vi "TestStep.vi"(7 "StrInit":string, 8 "error in":errorcluster caption="错误输入（无错误）", 9 "ParaIn":T2={"kCanBaud"=12, "DeviceType"=3, "DevInd"=0, "间隔延时"=0, "ID1(Hex)"="00000182", "DataIN1(Hex)"="000007d100000000", "DataRec1(Hex)"="000007d100000000", "ID2(Hex)"="00000182", "DataIN2(Hex)"="000007d100000000", "DataRec2(Hex)"="000007d100000000"} {"DeviceType" items=["PCI-CAN200"=7, "USB-CAN"=2, "USB-CAN200"=3]; "kCanBaud" items=["250k bps"=10, "10k bps"=2, "5k bps"=1, "50k bps"=5, "40k bps"=4, "20k bps"=3, "80k bps"=6, "100k bps"=7, "125k bps"=8, "200k bps"=9, "400k bps"=11, "500k bps"=12, "666k bps"=13, "800k bps"=14, "1000k bps"=15]}, 10 "ComStr":refnum<vi>, 11 "ComIn":refnum<visa-resource-name>) -> (0 "error out":errorcluster caption="错误输出", 1 "OK?":bool, 2 "通信？":bool, 3 "ComOut":refnum<visa-resource-name>, 4 "Time":u32, 5 "StrOut":string)   [LabVIEW 2013]
uses:
  USBCAN/DevType.ctl
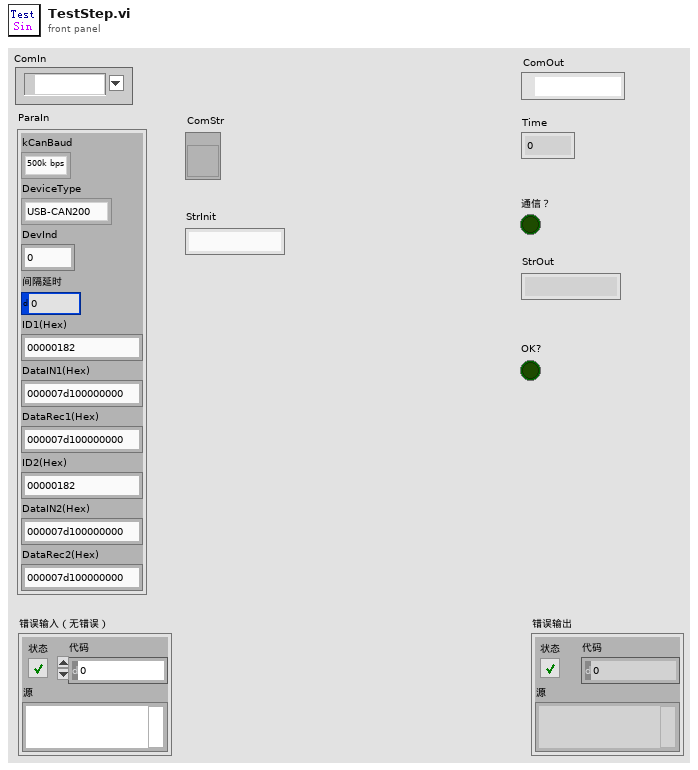
[diagram p1: front panel]
types:
  T1 = typedef "DevType.ctl" = u16
  T2 = cluster{"kCanBaud":u8, "DeviceType":T1, "DevInd":u16, "间隔延时":u32, "ID1(Hex)":string, "DataIN1(Hex)":string, "DataRec1(Hex)":string, "ID2(Hex)":string, "DataIN2(Hex)":string, "DataRec2(Hex)":string}
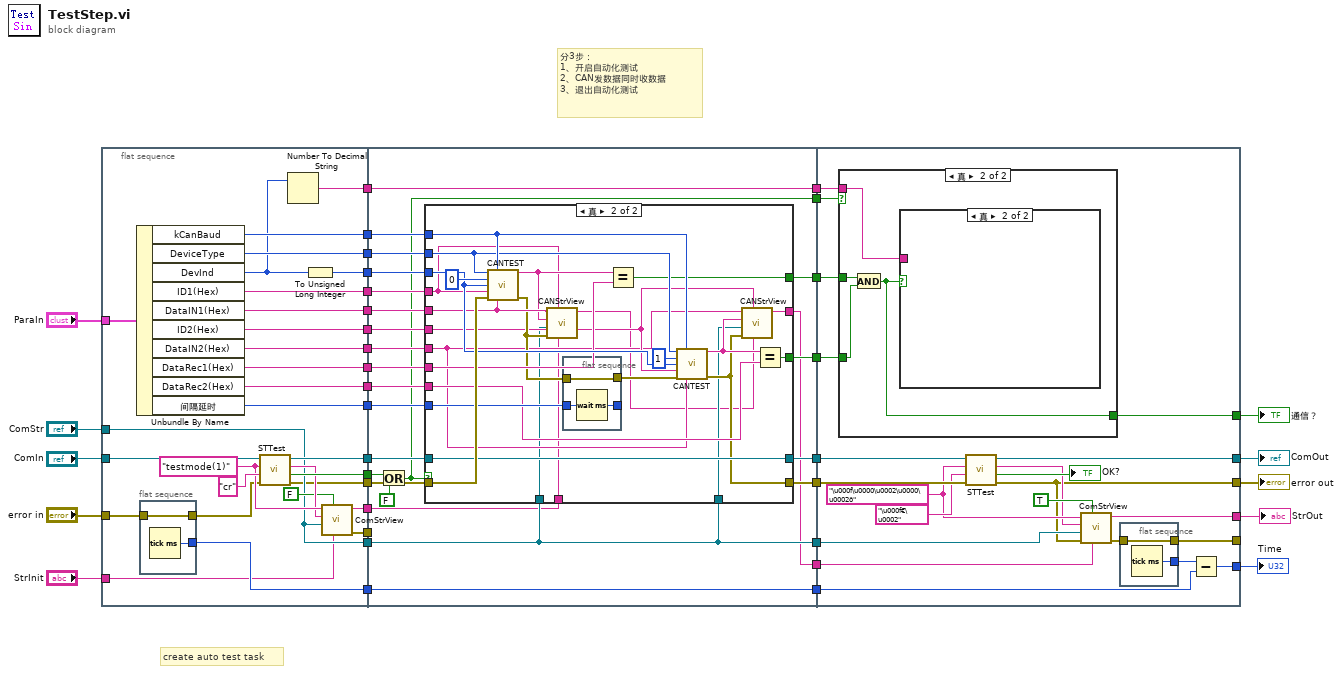
[diagram p0: block diagram]
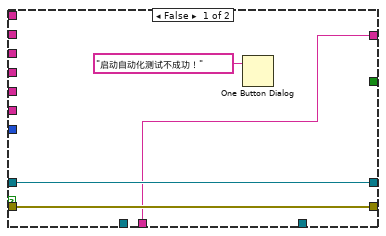
[diagram p2: hidden frame]
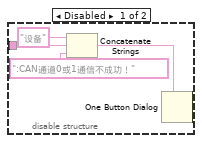
[diagram p5: hidden frame]
diagram:
  # "create auto test task"
  # "分3步：\n1、开启自动化测试\n2、CAN发数据同时收数据\n3、退出自动化测试"
  n1 = flat-sequence {
    tunnel: "ComIn" -> [w65]
    tunnel: "error in" -> [w41]
    tunnel: [w63] -> w35
    tunnel: [w38] -> w34
    tunnel: [w62] -> w33
    tunnel: "ParaIn" -> [w61]
    tunnel: [w60] -> w31
    tunnel: [w59] -> w30
    tunnel: [w49] -> w29
    tunnel: [w58] -> w28
    tunnel: [w57] -> w27
    tunnel: [w56] -> w26
    tunnel: [w55] -> w25
    tunnel: [w54] -> w24
    tunnel: [w53] -> w23
    tunnel: [w52] -> w22
    tunnel: [w50] -> w14
    tunnel: "ComStr" -> [w43]
    tunnel: [w46] -> w10
    tunnel: [w45] -> w9
    tunnel: [w43] -> w8
    tunnel: [w40] -> w6
    tunnel: "StrInit" -> [w39]
    tunnel: w35 -> [w79]
    tunnel: w34 -> [w91]
    tunnel: w33 -> [w72]
    tunnel: w31 -> [w87]
    tunnel: w30 -> [w86]
    tunnel: w29 -> [w85]
    tunnel: w28 -> [w89]
    tunnel: w27 -> [w84]
    tunnel: w26 -> [w90]
    tunnel: w25 -> [w83]
    tunnel: w24 -> [w88]
    tunnel: w23 -> [w82]
    tunnel: w22 -> [w81]
    tunnel: [w78] -> w21
    tunnel: [w80] -> w20
    tunnel: [w71] -> w18
    tunnel: [w77] -> w17
    tunnel: [w76] -> w16
    tunnel: [w75] -> w15
    tunnel: w14 -> [w75]
    tunnel: w10 -> [w69]
    tunnel: w9 -> [_]
    tunnel: w8 -> [w74]
    tunnel: [w74] -> w7
    tunnel: w6 -> [w70]
    tunnel: [w70] -> w5
    tunnel: [w68] -> w3
    tunnel: w21 -> [w146]
    tunnel: w20 -> [w145]
    tunnel: [w144] -> w13
    tunnel: [w125] -> w19
    tunnel: w18 -> [w143]
    tunnel: w17 -> [w142]
    tunnel: w16 -> [w141]
    tunnel: w15 -> [w140]
    tunnel: [w139] -> w12
    tunnel: [w133] -> w2
    tunnel: w7 -> [w132]
    tunnel: [w130] -> _
    tunnel: w5 -> [w128]
    tunnel: [w127] -> w4
    tunnel: w3 -> [w126]
    frame #0 {
      w48 = "testmode(1)" ("CMDIn")
      n2 = Unbundle By Name(w61) -> ("kCanBaud"=w60:u8, "DeviceType"=w59:T1, "DevInd"=w51:u16, "ID1(Hex)"=w56:string, "DataIN1(Hex)"=w58:string, "ID2(Hex)"=w57:string, "DataIN2(Hex)"=w55:string, "DataRec1(Hex)"=w53:string, "DataRec2(Hex)"=w52:string, "间隔延时"=w54:u32)
      n3 = flat-sequence {
        tunnel: [w67] -> w42
        tunnel: w41 -> [w67]
        tunnel: [w66] -> w40
        frame #0 {
          n4 = Tick Count (ms)() -> (millisecond timer value=w66:u32)
        }
      }
      n5 = call "STTest.vi"("error in"=w42, "React"="cr", "CMDIn"=w48, "ComIn"=w65) -> ("error out"=w38:errorcluster, "OK?"=w62:bool, "ReactStr"=w47:string, "ComOut"=w63:refnum<visa-resource-name>)  [unwired: 4 in]
      n6 = Number To Decimal String(number=w51) -> (decimal integer string=w50:string)  [unwired: 1 in]
      n7 = To Unsigned Long Integer(number=w51) -> (unsigned 32bit integer=w49:u32)
      n8 = call "ComStrView.vi"("StrInit"=w39, "Hex？"=FALSE, "ComConn"=w43, "ReactStrIn"=w47, "CMDIn"=w48) -> ("error out"=w45:errorcluster, "连接字符串显示"=w46:string)  [unwired: 5 in]
    }
    frame #1 {
      n9 = Or(x=w72, y=FALSE) -> (x .or. y?=w71:bool)
      n10 = case shown="真" w71 {
        tunnel: w91 -> [w95 w121]
        tunnel: w90 -> [_ w106]
        tunnel: w89 -> [_ w108]
        tunnel: w88 -> [_ w119]
        tunnel: w87 -> [_ w117]
        tunnel: w86 -> [_ w116]
        tunnel: w85 -> [_ w114]
        tunnel: w84 -> [_ w104]
        tunnel: w83 -> [_ w103]
        tunnel: w82 -> [_ w113]
        tunnel: w81 -> [_ w112]
        tunnel: [w95 w101] -> w80
        tunnel: w79 -> [w94 w111]
        tunnel: [w94 w111] -> w78
        tunnel: [_ w110] -> w77
        tunnel: [_ w109] -> w76
        tunnel: w74 -> [_ w100]
        tunnel: w74 -> [_ w99]
        tunnel: w69 -> [w92 w98]
        tunnel: [w92 w96] -> w68
        frame False {
          n11 = One Button Dialog(message="启动自动化测试不成功！" ("消息")) -> ()  [unwired: 1 in, 1 out]
        }
        frame True {
          n12 = call "CANTEST.vi"("DeviceType"=w116, "kCanBaud"=w117, "CANChannel"=u32 0, "DevInd"=w114, "ID(Hex 高位有效)"=w106, "错误输入"=w121, "Data Input(Hex)"=w108) -> ("帧数据"=w107:string, "错误输出"=w105:errorcluster)  [unwired: 5 in, 2 out]
          n13 = call "CANStrView.vi"("StrInit"=w98, "ID"=w106, "error in"=w105, "CANStrView"=w100, "DataRec"=w107, "DataTrans"=w108) -> ("连接显示"=w97:string)  [unwired: 4 in, 1 out]
          n14 = flat-sequence {
            tunnel: w105 -> [w122]
            tunnel: w119 -> [w124]
            tunnel: [w123] -> _
            tunnel: [w122] -> w118
            frame #0 {
              n15 = Wait (ms)(milliseconds to wait=w124) -> (millisecond timer value=w123:u32)
            }
          }
          n16 = Equal?(x=w107, y=w113) -> (x = y?=w110:bool)
          n17 = call "CANTEST.vi"("DeviceType"=w116, "kCanBaud"=w117, "CANChannel"=u32 1, "DevInd"=w114, "ID(Hex 高位有效)"=w104, "错误输入"=w118, "Data Input(Hex)"=w103) -> ("帧数据"=w102:string, "错误输出"=w101:errorcluster)  [unwired: 5 in, 2 out]
          n18 = call "CANStrView.vi"("StrInit"=w97, "ID"=w104, "error in"=w101, "CANStrView"=w99, "DataRec"=w102, "DataTrans"=w103) -> ("连接显示"=w96:string)  [unwired: 4 in, 1 out]
          n19 = Equal?(x=w102, y=w112) -> (x = y?=w109:bool)
        }
      }
    }
    frame #2 {
      w136 = "\u000f\u0000\u0002\u0000\u0002ð"
      n20 = case shown="真" w143 {
        tunnel: w142 -> [_ w152]
        tunnel: w141 -> [_ w151]
        tunnel: w140 -> [_ w150]
        tunnel: [_ w149] -> w139
        frame False {
        }
        frame True {
          n21 = And(x=w152, y=w151) -> (x .and. y?=w149:bool)
          n22 = case shown="真" w149 {
            tunnel: w150 -> [w153 _]
            frame False {
              n23 = disable-structure shown="启用" {
                disable-tunnel: w153 -> [w156 _]
                frame Disabled {
                  n24 = Concatenate Strings("设备", w156, ":CAN通道0或1通信不成功！") -> (w154:string)
                  n25 = One Button Dialog(message=w154) -> ()  [unwired: 1 in, 1 out]
                }
                frame Enabled {
                }
              }
            }
            frame True {
            }
          }
        }
      }
      n26 = call "STTest.vi"("error in"=w145, "React"="\u000f€\u0002", "CMDIn"=w136, "ComIn"=w146) -> ("error out"=w125:errorcluster, "OK?"=→"OK?":bool, "ReactStr"=w134:string, "ComOut"=w144:refnum<visa-resource-name>)  [unwired: 4 in]
      n27 = call "ComStrView.vi"("StrInit"=w126, "Hex？"=TRUE, "error in"=w125, "ComConn"=w132, "ReactStrIn"=w134, "CMDIn"=w136) -> ("error out"=w131:errorcluster, "连接字符串显示"=w133:string)  [unwired: 4 in]
      n28 = flat-sequence {
        tunnel: w131 -> [w148]
        tunnel: [w148] -> w130
        tunnel: [w147] -> w129
        frame #0 {
          n29 = Tick Count (ms)() -> (millisecond timer value=w147:u32)
        }
      }
      n30 = Subtract(x=w129, y=w128) -> (x-y=w127:u32)
    }
  }
  "error out" <- w19
  "ComOut" <- w13
  "通信？" <- w12
  "Time" <- w4
  "StrOut" <- w2
